vi "Communication - Heartbeat (FGV).vi"(7 "Action":T1=enum."Write", 8 "error in (no error)":errorcluster, 9 "Previous":string[](array[string]), 10 "Timestamp":string[](array[string]), 11 "IP":string[](array[string])) -> (0 "error out":errorcluster, 1 "Previous Out":string[](array[string]), 2 "Timestamp Out":string[](array[string]), 3 "IP Out":string[](array[string]))   [LabVIEW 2019]
uses:
  Controls/FGV States.ctl
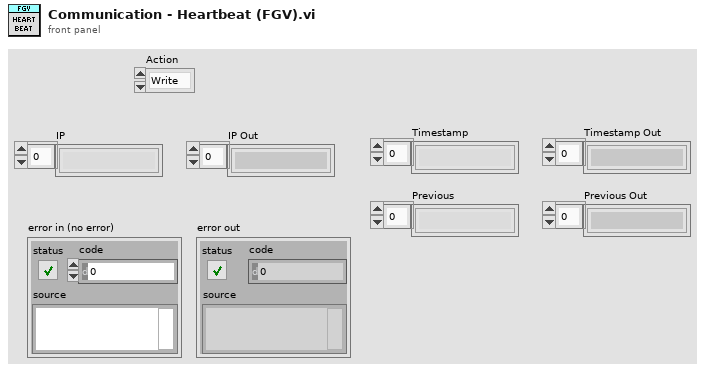
[diagram p1: front panel]
types:
  T1 = typedef "FGV States.ctl" = enum16{"Read", "Write"}
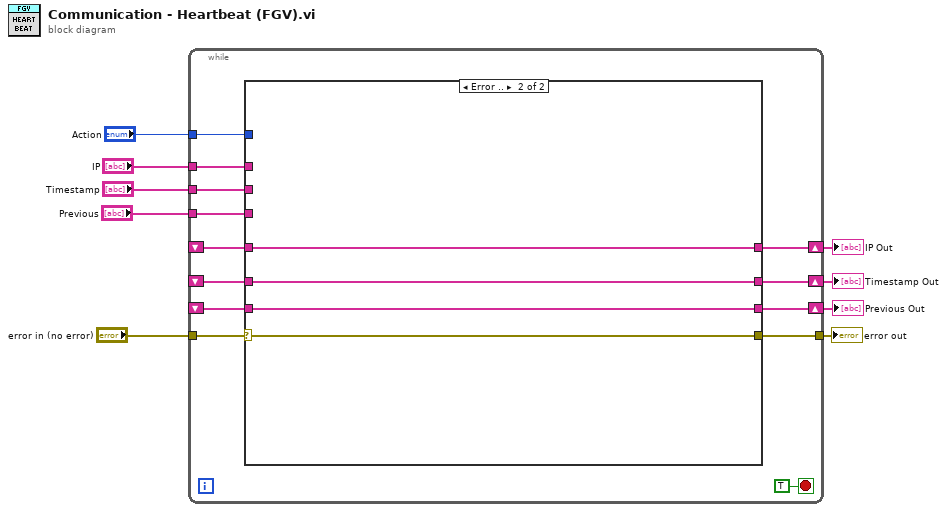
[diagram p0: block diagram]
diagram:
  n1 = while {
    tunnel: "Action" -> [w22]
    tunnel: "IP" -> [w20]
    shift-right: [w21] -> w7
    shift-left: _ -> [w19]
    tunnel: "error in (no error)" -> [w17]
    tunnel: [w16] -> w5
    tunnel: "Timestamp" -> [w14]
    shift-right: [w15] -> w4
    shift-left: _ -> [w13]
    tunnel: "Previous" -> [w11]
    shift-right: [w12] -> w1
    shift-left: _ -> [w10]
    stop <- TRUE stop-if-true
    n2 = case shown="Error .." w17 {
      selector: w17 -> [w29 w45]
      tunnel: w22 -> [w34 _]
      tunnel: [w33 w46] -> w21
      tunnel: w20 -> [w32 _]
      tunnel: w19 -> [w31 w46]
      tunnel: [w30 w45] -> w16
      tunnel: [w28 w44] -> w15
      tunnel: w14 -> [w27 _]
      tunnel: w13 -> [w26 w44]
      tunnel: [w25 w43] -> w12
      tunnel: w11 -> [w24 _]
      tunnel: w10 -> [w23 w43]
      frame No Error {
        n3 = case shown="\"Read\", Default" w34 {
          tunnel: [w38 w42] -> w33
          tunnel: w32 -> [_ w42]
          tunnel: w31 -> [w38 _]
          tunnel: [w37 w41] -> w30
          tunnel: w29 -> [w37 w41]
          tunnel: [w36 w40] -> w28
          tunnel: w27 -> [_ w40]
          tunnel: w26 -> [w36 _]
          tunnel: [w35 w39] -> w25
          tunnel: w24 -> [_ w39]
          tunnel: w23 -> [w35 _]
          frame "Read", Default {
          }
          frame "Write" {
          }
        }
      }
      frame Error {
      }
    }
  }
  "IP Out" <- w7
  "error out" <- w5
  "Timestamp Out" <- w4
  "Previous Out" <- w1
